vi "Configurable Graph.vi"(6 "A":dbl, 7 "B":dbl, 10 "Instrument Label":string, 11 "Port #":dbl) -> (2 "Scaled output":dbl)   [LabVIEW 2020]
panel:
  in  "Input Voltages":dbl[](array[numeric])
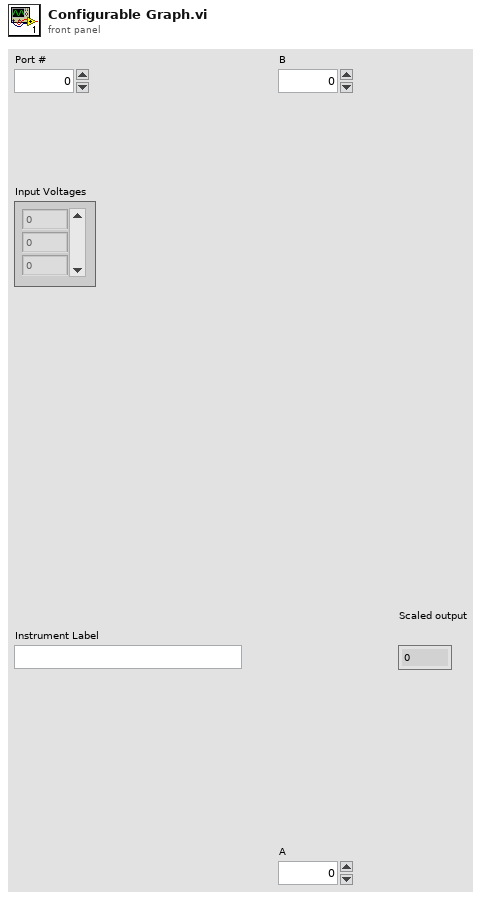
[diagram p1: front panel]
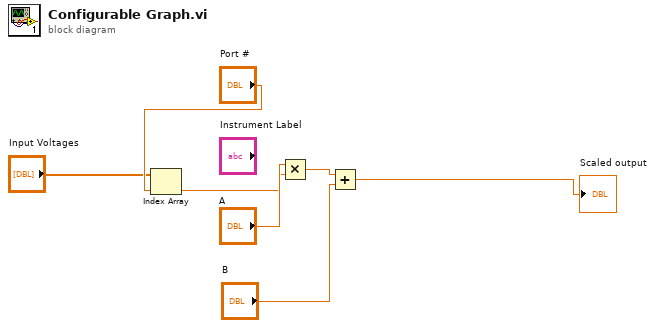
[diagram p0: block diagram]
diagram:
  n1 = Index Array(array="Input Voltages", index="Port #") -> (element=w2:dbl)
  n2 = Multiply(x="A", y=w2) -> (x*y=w4:dbl)
  n3 = Add(x=w4, y="B") -> (x+y=→"Scaled output":dbl)
